vi "Average(Recursive).vi"(10 "DataInput":dbl) -> (2 "Average":dbl)   [LabVIEW 2020]
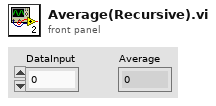
[diagram p1: front panel]
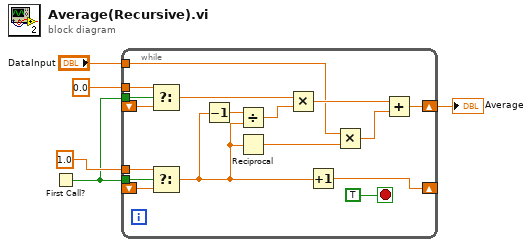
[diagram p0: block diagram]
diagram:
  n1 = First Call?() -> (First Call?: T/F=w2:bool)
  n2 = while {
    tunnel: "DataInput" -> [w18]
    shift-right: [w17] -> w4
    shift-left: _ -> [w9]
    shift-right: [w10] -> _
    shift-left: _ -> [w11]
    tunnel: w2 -> [w14]
    tunnel: 1.0 -> [w12]
    tunnel: w2 -> [w8]
    tunnel: 0.0 -> [w7]
    stop <- TRUE stop-if-true
    n3 = Select(t=w7, s=w8, f=w9) -> (s? t:f=w6:dbl)
    n4 = Select(t=w12, s=w14, f=w11) -> (s? t:f=w13:dbl)
    n5 = Decrement(x=w13) -> (x-1=w15:dbl)
    n6 = Divide(x=w15, y=w13) -> (x/y=w22:dbl)
    n7 = Reciprocal(x=w13) -> (1/x=w21:dbl)
    n8 = Multiply(x=w6, y=w22) -> (x*y=w20:dbl)
    n9 = Increment(x=w13) -> (x+1=w10:dbl)
    n10 = Multiply(x=w18, y=w21) -> (x*y=w19:dbl)
    n11 = Add(x=w20, y=w19) -> (x+y=w17:dbl)
  }
  "Average" <- w4
